vi "Idx_calc.vi"(1 "bit4":u8, 2 "bit3":u8) -> (0 "idx":u8)   [LabVIEW 2017]
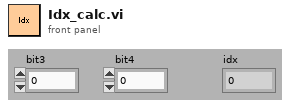
[diagram p1: front panel]
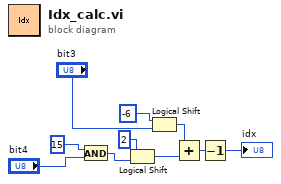
[diagram p0: block diagram]
diagram:
  n1 = And(x=u8 15, y="bit4") -> (x .and. y?=w4:u8)
  n2 = Logical Shift(y=i8 2, x=w4) -> (x << y=w3:u8)
  n3 = Logical Shift(y=i8 -6, x="bit3") -> (x << y=w9:u8)
  n4 = Add(x=w9, y=w3) -> (x+y=w10:u8)
  n5 = Decrement(x=w10) -> (x-1=→"idx":u8)
